vi "Change Comparison Algorithm.vi"(5 "Type":T1, 6 "VI Path":path, 7 "Operation":string, 8 "error in (no error)":errorcluster) -> (0 "error out":errorcluster)   [LabVIEW 2017]
doc: "Updates the comparison algorithm to use a more complex one for floating point equal/not equal comparisons"
uses:
  <vilib>/Utility/Data Type/Type Definitions/Data Type.ctl
  <vilib>/Utility/traverseref.llb/TRef TravTarget.ctl
  <vilib>/Utility/traverseref.llb/VI Scripting - Traverse.lvlib
  <vilib>/Utility/Data Type/NI_Data Type.lvlib
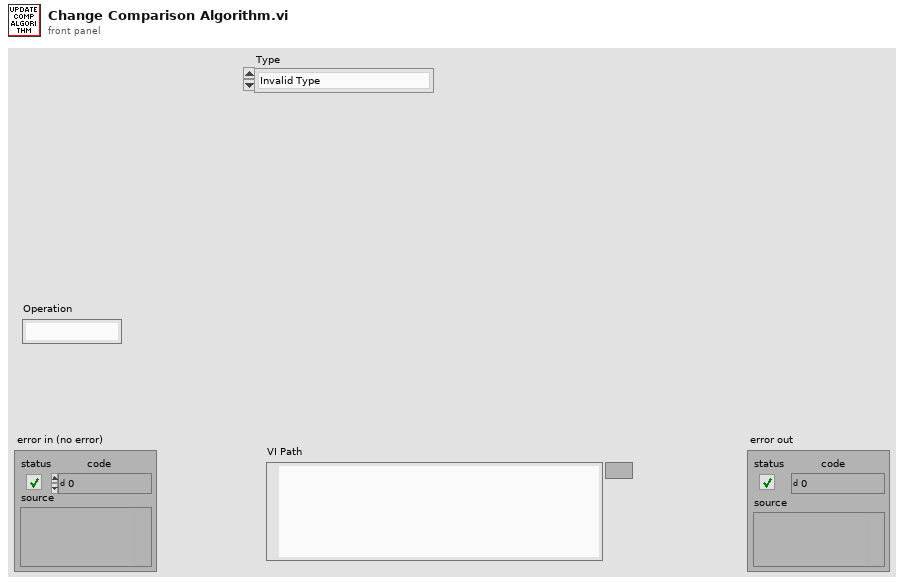
[diagram p1: front panel]
types:
  T1 = typedef "NI_Data Type.lvlib/Data Type.ctl" = enum8{"Invalid Type", "Void", "I8", "I16", "I32", "I64", "U8", "U16", "U32", "U64", "Single Float", "Double Float", "Extended Float", "Single Complex", "Double Complex", "Extended Complex", "Enum U8", "Enum U16", "Enum U32", "Enum U64", "Single Float With Unit", "Double Float With Unit", "Extended Float With Unit", "Single Complex with Unit", "Double Complex with Unit", "Extended Complex with Unit", "Boolean", "String", "Path", "Picture", "Tag", "Array", "Cluster", "Variant", "LV Variant", "Waveform", "Timestamp", "Digital Waveform", "Digital Data", "ExpressData", "Refnum", "External Data", "VI", "Poly VI", "LabVIEW Class Instance", "Fixed Point"}
  T2 = typedef "TRef TravTarget.ctl" = enum16{"FP", "BD", "Other"}
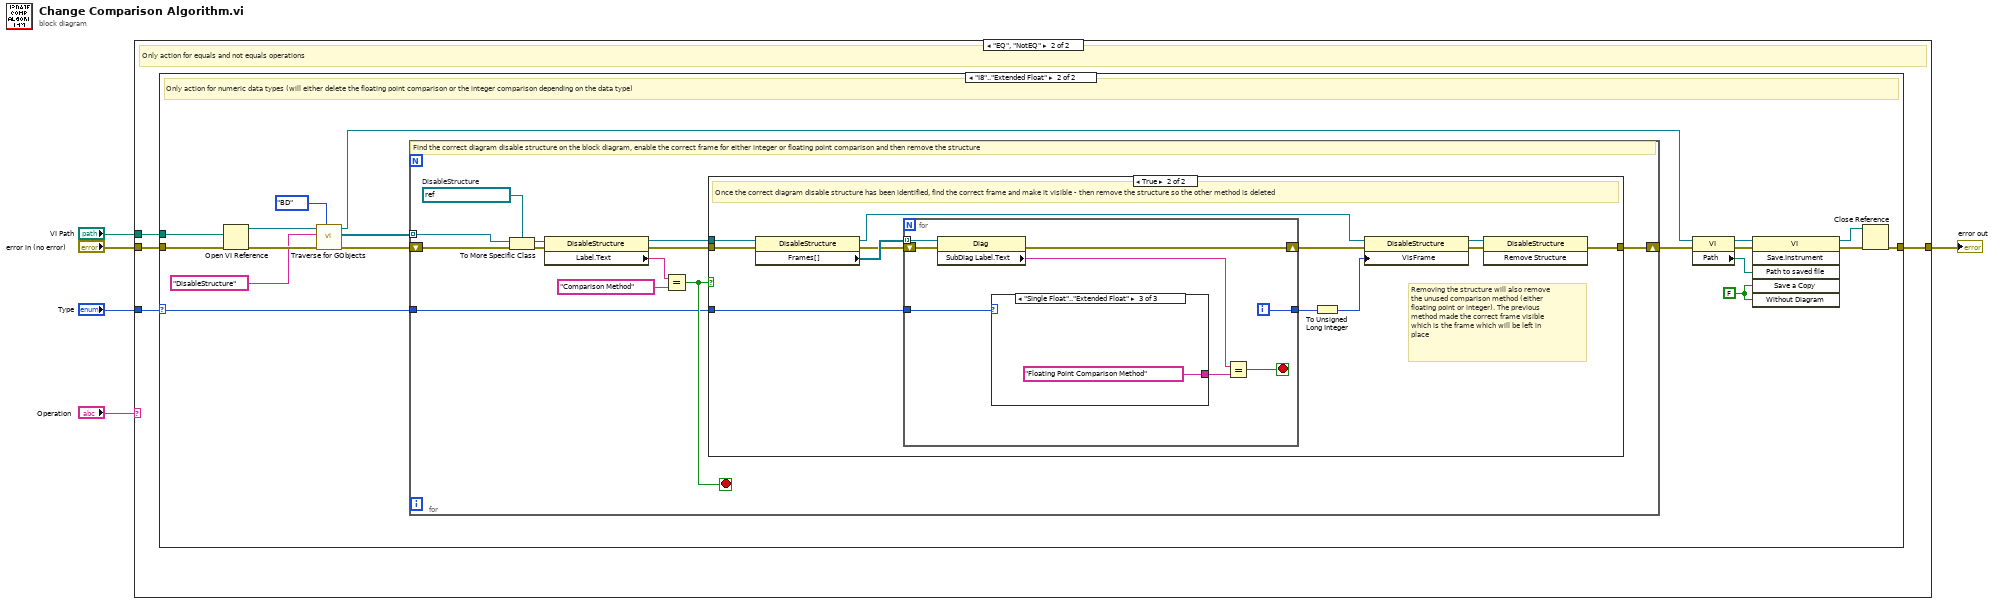
[diagram p0: block diagram]
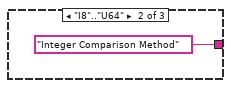
[diagram p6: hidden frame]
diagram:
  n1 = case shown="\"EQ\", \"NotEQ\"" "Operation" {
    tunnel: [w6 w10] -> w5
    tunnel: "error in (no error)" -> [w6 w9]
    tunnel: "VI Path" -> [_ w8]
    tunnel: "Type" -> [_ w7]
    frame Default {
    }
    frame "EQ", "NotEQ" {
      # "Only action for equals and not equals operations"
      n2 = case shown="\"I8\"..\"Extended Float\"" w7 {
        selector: w7 -> [_ w14]
        tunnel: [w11 w12] -> w10
        tunnel: w9 -> [w11 w16]
        tunnel: w8 -> [_ w15]
        frame "Invalid Type", Default {
        }
        frame "I8".."Extended Float" {
          w17 = FALSE ("Save a Copy")
          # "Only action for numeric data types (will either delete the floating point comparison or the integer comparison depending on the data type)"
          n3 = Open VI Reference(vi path=w15, error in (no error)=w16) -> (vi reference=w26:refnum<vi>, error out=w28:errorcluster)  [unwired: 4 in]
          n4 = call <vilib>:"Traverse for GObjects.vi"("Traverse Target"=TRef_TravTarget."BD", "error in (no error)"=w28, "Class Name"="DisableStructure", "VI Refnum"=w26) -> ("error out"=w27:errorcluster, "References"=w23:refnum<vi>[], "dup VI Refnum"=w19:refnum<vi>)  [unwired: 4 in, 1 out]
          n5 = for {
            tunnel: w23 -> [w41] mode=indexing
            shift-right: [w38] -> w29
            shift-left: w27 -> [w39]
            tunnel: w14 -> [w30]
            stop <- w40 stop-if-true
            w37 = refnum<vi> refnum  # DisableStructure
            # "Find the correct diagram disable structure on the block diagram, enable the correct frame for either integer or floating point comparison and then remove the structure"
            n6 = To More Specific Class(target class=w37, reference=w41, error in=w39) -> (specific class reference=w36:refnum<vi>, error out=w33:errorcluster)
            n7 = property class="DisableStructure"(reference=w36, error in=w33) -> (reference out=w34:refnum<vi>, error out=w32:errorcluster, "Label.Text"=w35:string)
            n8 = Equal?(x=w35, y="Comparison Method") -> (x = y?=w40:bool)
            n9 = case shown="True" w40 {
              tunnel: w34 -> [_ w54]
              tunnel: w32 -> [w42 w53]
              tunnel: [w42 w44] -> w38
              tunnel: w30 -> [_ w51]
              frame False {
              }
              frame True {
                # "Removing the structure will also remove the unused comparison method (either floating point or integer). The previous method made the correct frame visible which is the frame which will be left in place"
                # "Once the correct diagram disable structure has been identified, find the correct frame and make it visible - then remove the structure so the other method is deleted"
                n10 = property class="DisableStructure"(reference=w54, error in=w53) -> (reference out=w49:refnum<vi>, error out=w50:errorcluster, "Frames[]"=w52:refnum<vi>[])
                n11 = for {
                  tunnel: w52 -> [w62] mode=indexing
                  tunnel: w51 -> [w56]
                  shift-right: [w58] -> w48
                  shift-left: w50 -> [w59]
                  tunnel: [w55] -> w47
                  i -> [w55]
                  stop <- w57 stop-if-true
                  n12 = property class="Diag"(reference=w62, error in=w59) -> (error out=w58:errorcluster, "SubDiag Label.Text"=w60:string)  [unwired: 1 out]
                  n13 = case shown="\"Single Float\"..\"Extended Float\"" w56 {
                    tunnel: [_ "Integer Comparison Method" ("y") "Floating Point Comparison Method" ("y")] -> w61
                    frame Default {
                    }
                    frame "I8".."U64" {
                    }
                    frame "Single Float".."Extended Float" {
                    }
                  }
                  n14 = Equal?(x=w60, y=w61) -> (x = y?=w57:bool)
                }
                n15 = To Unsigned Long Integer(number=w47) -> (unsigned 32bit integer=w43:u32)
                n16 = property class="DisableStructure"(reference=w49, error in=w48, "VisFrame"=w43) -> (reference out=w46:refnum<vi>, error out=w45:errorcluster)
                n17 = invoke class="DisableStructure" method="Remove Structure"(reference=w46, error in=w45) -> (error out=w44:errorcluster)  [unwired: 1 in, 2 out]
              }
            }
          }
          n18 = property class="VI"(reference=w19, error in=w29) -> (reference out=w18:refnum<vi>, error out=w20:errorcluster, "Path"=w13:path)
          n19 = invoke class="VI" method="Save.Instrument"(reference=w18, error in=w20, "Path to saved file"=w13, "Save a Copy"=w17, "Without Diagram"=w17) -> (reference out=w21:refnum<vi>, error out=w22:errorcluster)  [unwired: 1 in, 4 out]
          n20 = Close Reference(reference=w21, error in (no error)=w22) -> (error out=w12:errorcluster)
        }
      }
    }
  }
  "error out" <- w5
